vi "Configure Hardware.vi"(8 "error in (no error)":errorcluster, 11 "Hardware Resources in":T1={"DAQmx Channel 1"="", "DAQmx Channel 2"="", "DAQmx Channel 3"="", "Channel 1 Name"="Battery Voltage", "Channel 2 Name"="Battery Current", "Channel 3 Name"="Brake torque", "Input Config Channel 1"=-1, "Input Config Channel 2"=-1, "Input Config Channel 3"=-1, "Offset Channel 1"=0.0, "Offset Channel 2"=0.0, "Offset Channel 3"=0.0, "Scale Channel 1"=0.0, "Scale Channel 2"=0.0, "Scale Channel 3"=0.0, "Sample time"=50, "Samples per second"=1000.0, "Sample mode"=10123, "Samples per channel"=0, "DAQmx AI Task"="", "DAQmx Channel 4"="", "Channel 3 Name 2"="", "Input Config Channel 4"=-1, "Offset Channel 4"=0.0, "Scale Channel 4"=0.0} {"Input Config Channel 4" items=["Default"=-1, "RSE"=10083, "NRSE"=10078, "Differential"=10106, "Pseudodifferential"=12529]; "Input Config Channel 3" items=["Default"=-1, "RSE"=10083, "NRSE"=10078, "Differential"=10106, "Pseudodifferential"=12529]; "Input Config Channel 2" items=["Default"=-1, "RSE"=10083, "NRSE"=10078, "Differential"=10106, "Pseudodifferential"=12529]; "Input Config Channel 1" items=["Default"=-1, "RSE"=10083, "NRSE"=10078, "Differential"=10106, "Pseudodifferential"=12529]; "Sample mode" items=["Hardware Timed Single Point"=12522, "Finite Samples"=10178, "Continuous Samples"=10123]}) -> (0 "error out":errorcluster, 3 "Hardware Resources out":T1={"DAQmx Channel 1"="", "DAQmx Channel 2"="", "DAQmx Channel 3"="", "Channel 1 Name"="Battery Voltage", "Channel 2 Name"="Battery Current", "Channel 3 Name"="Brake torque", "Input Config Channel 1"=-1, "Input Config Channel 2"=-1, "Input Config Channel 3"=-1, "Offset Channel 1"=0.0, "Offset Channel 2"=0.0, "Offset Channel 3"=0.0, "Scale Channel 1"=0.0, "Scale Channel 2"=0.0, "Scale Channel 3"=0.0, "Sample time"=50, "Samples per second"=1000.0, "Sample mode"=0, "Samples per channel"=0, "DAQmx AI Task"="", "DAQmx Channel 4"="", "Channel 3 Name 2"="", "Input Config Channel 4"=-1, "Offset Channel 4"=0.0, "Scale Channel 4"=0.0} {"Input Config Channel 4" items=["Default"=-1, "RSE"=10083, "NRSE"=10078, "Differential"=10106, "Pseudodifferential"=12529]; "Input Config Channel 3" items=["Default"=-1, "RSE"=10083, "NRSE"=10078, "Differential"=10106, "Pseudodifferential"=12529]; "Input Config Channel 2" items=["Default"=-1, "RSE"=10083, "NRSE"=10078, "Differential"=10106, "Pseudodifferential"=12529]; "Input Config Channel 1" items=["Default"=-1, "RSE"=10083, "NRSE"=10078, "Differential"=10106, "Pseudodifferential"=12529]; "Sample mode" items=["Hardware Timed Single Point"=12522, "Finite Samples"=10178, "Continuous Samples"=10123]})   [LabVIEW 2018, in "Acquisition.lvlib"]
doc: "Configure the hardware."
uses:
  Acquisition.lvlib
  Hardware Configuration.ctl
  <vilib>/DAQmx/configure/timing.llb/DAQmx Timing (Sample Clock).vi
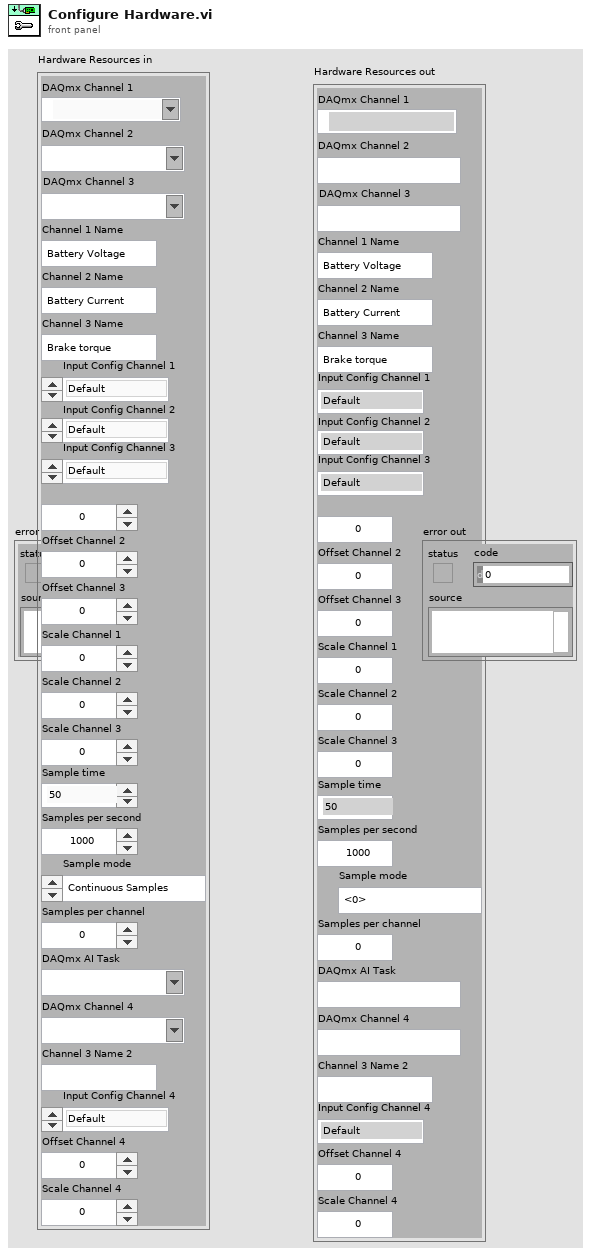
[diagram p1: front panel]
types:
  T1 = typedef "Acquisition.lvlib/Hardware Configuration.ctl" = cluster{"DAQmx Channel 1":tag, "DAQmx Channel 2":tag, "DAQmx Channel 3":tag, "Channel 1 Name":string, "Channel 2 Name":string, "Channel 3 Name":string, "Input Config Channel 1":i32, "Input Config Channel 2":i32, "Input Config Channel 3":i32, "Offset Channel 1":dbl, "Offset Channel 2":dbl, "Offset Channel 3":dbl, "Scale Channel 1":dbl, "Scale Channel 2":dbl, "Scale Channel 3":dbl, "Sample time":u32, "Samples per second":dbl, "Sample mode":u16, "Samples per channel":i32, "DAQmx AI Task":refnum<k21>, "DAQmx Channel 4":tag, "Channel 3 Name 2":string, "Input Config Channel 4":i32, "Offset Channel 4":dbl, "Scale Channel 4":dbl}
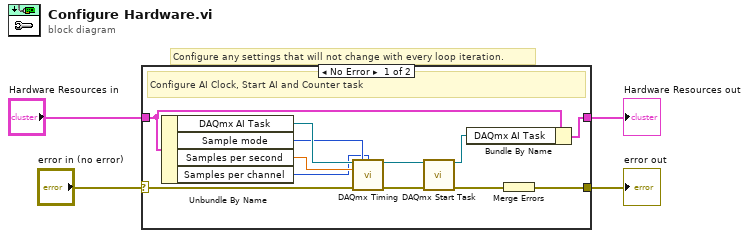
[diagram p0: block diagram]
diagram:
  # "Configure any settings that will not change with every loop iteration."
  n1 = case shown="No Error" "error in (no error)" {
    selector: "error in (no error)" -> [w7 w17]
    tunnel: [w6 w17] -> w3
    tunnel: "Hardware Resources in" -> [w15 w18]
    tunnel: [w16 w18] -> w1
    frame No Error {
      # "Configure AI Clock, Start AI and Counter task"
      n2 = Unbundle By Name(w15) -> ("DAQmx AI Task"=w12:refnum<k21>, "Sample mode"=w10:u16, "Samples per second"=w9:dbl, "Samples per channel"=w8:i32)
      n3 = call-poly <vilib>:"DAQmx Timing.vi"("task/channels in"=w12, "sample mode"=w10, "samples per channel"=w8, "rate"=w9, "error in"=w7) -> ("task out"=w11:refnum<k21>, "error out"=w13:errorcluster)  [unwired: 9 in]
      n4 = call <vilib>:"DAQmx Start Task.vi"("task/channels in"=w11, "error in"=w13) -> ("task out"=w14:refnum<k21>, "error out"=w5:errorcluster)  [unwired: 12 in]
      n5 = Bundle By Name(cluster=w15, "DAQmx AI Task"=w14) -> (w16:T1)
      n6 = Merge Errors(w5) -> (w6:errorcluster)
    }
    frame Error {
    }
  }
  "Hardware Resources out" <- w1
  "error out" <- w3
